vi "FRCts20_WebMethods_Division_DELETE.vi"(7 "httpRequestID":u32, 10 "division":string, 11 "competition":string) -> ()   [LabVIEW 2014, in "FRCts20_WebMethods.lvlib"]
doc: "<B>DELETE</B> the specified <B>division</B> resource\n\nhttp://<server address>:<port>/FRCts/competition/<B>competition</B>/division/<B>division</B>\n\n{requires authentication}"
uses:
  FRCts20_WebMethods.lvlib
  <vilib>/wsapi/NI_WebServices.lvlib
  Backend/source/VI Source/FRCts20_Backend_API/FRCts20_Backend_API_SW.ctl
  Backend/source/VI Source/FRCts20_Backend_API/FRCts20_Backend_API.lvlib
  Backend/source/VI Source/FRCts20_Backend_API/FRCts20_Backend_API_Status.ctl
  Backend/source/VI Source/FRCts20_Backend_API/FRCts20_Backend_API_Division.ctl
  Backend/source/VI Source/FRCts20_Backend_API/FRCts20_Backend_API_Command_Division.ctl
  Backend/source/VI Source/FRCts20_Backend_API/FRCts20_Backend_API_Application.vi
panel:
  in  "query":string
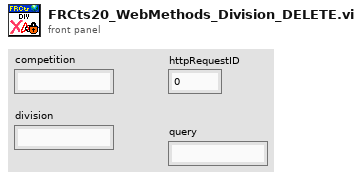
[diagram p1: front panel]
types:
  T1 = typedef "FRCts20_Backend_API.lvlib/FRCts20_Backend_API_Command_Division.ctl" = string
  T2 = typedef "FRCts20_Backend_API.lvlib/FRCts20_Backend_API_Division.ctl" = cluster{"Location":string, "Team":u32[], "APIReturn":string, "RootCmd":enum16{"Issues", "Software", "All"}, "SWType":T3, "Status":T4, "Competition":string}
  T3 = typedef "FRCts20_Backend_API.lvlib/FRCts20_Backend_API_SW.ctl" = string
  T4 = typedef "FRCts20_Backend_API.lvlib/FRCts20_Backend_API_Status.ctl" = enum16{"Open", "In Work", "Closed"}
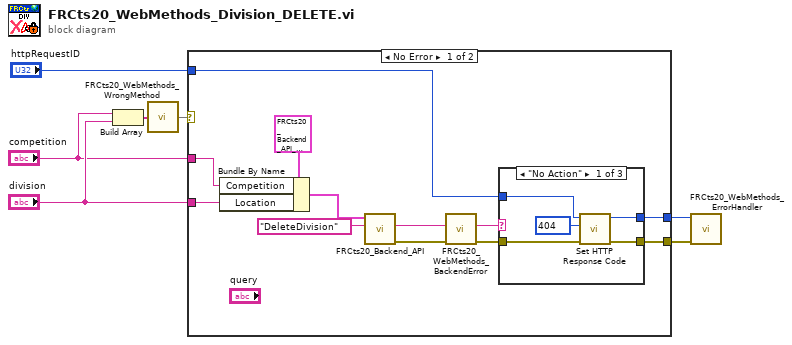
[diagram p0: block diagram]
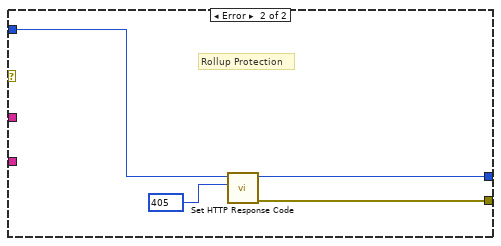
[diagram p4: hidden frame]
diagram:
  n1 = Build Array("competition", "division") -> (w6:string[])
  n2 = call "FRCts20_WebMethods_WrongMethod.vi"(4:w6) -> (1:w7)  [unwired: 3 in, 1 out]
  n3 = case shown="No Error" w7 {
    tunnel: "httpRequestID" -> [w9 w32]
    tunnel: [w8 w30] -> w3
    tunnel: [w10 w29] -> w4
    tunnel: "division" -> [w18 _]
    tunnel: "competition" -> [w17 _]
    frame No Error {
      n4 = Bundle By Name(cluster=T2 {"Location"="", "Team"=[], "APIReturn"="", "RootCmd"=enum."Issues", "SWType"="", "Status"=enum."Open", "Competition"=""} ("Division"), "Competition"=w17, "Location"=w18) -> (w16:T2)
      n5 = call-poly "FRCts20_Backend_API.vi"("Command"=T1 "DeleteDivision", 11:w16) -> ("error out"=w14:errorcluster, "Status"=w13:string)  [unwired: 7 in, 1 out]
      n6 = call "FRCts20_WebMethods_BackendError.vi"("error in (no error)"=w14, "Status"=w13) -> ("error out"=w11:errorcluster, "Status out"=w12:string)  [unwired: 8 in]
      n7 = case shown="\"No Action\"" w12 {
        tunnel: w11 -> [w21 w26 w28]
        tunnel: [w24 w26 w28] -> w10
        tunnel: w9 -> [w22 w25 w27]
        tunnel: [w23 w25 w27] -> w8
        frame "No Action" {
          w20 = 404 items=["100"=100, "101"=101, "200"=200, "201"=201, "202"=202, "203"=203, "204"=204, "205"=205, "206"=206, "300"=300, "301"=301, "302"=302, "303"=303, "304"=304, "305"=305, "306"=306, "307"=307, "400"=400, "401"=401, "402"=402, "403"=403, "404"=404, "405"=405, "406"=406, "407"=407, "408"=408, "409"=409, "410"=410, "411"=411, "412"=412, "413"=413, "414"=414, "415"=415, "416"=416, "417"=417, "500"=500, "501"=501, "502"=502, "503"=503, "504"=504, "505"=505] ("response code (200)")
          n8 = call <vilib>:"Set HTTP Response Code.vi"("error in (no error)"=w21, "response code (200)"=w20, "httpRequestID"=w22) -> ("error out"=w24:errorcluster, "httpRequestID out"=w23:u32)  [unwired: 7 in]
        }
        frame "Backend Error", Default {
        }
        frame "Success" {
        }
      }
    }
    frame Error {
      w31 = 405 items=["100"=100, "101"=101, "200"=200, "201"=201, "202"=202, "203"=203, "204"=204, "205"=205, "206"=206, "300"=300, "301"=301, "302"=302, "303"=303, "304"=304, "305"=305, "306"=306, "307"=307, "400"=400, "401"=401, "402"=402, "403"=403, "404"=404, "405"=405, "406"=406, "407"=407, "408"=408, "409"=409, "410"=410, "411"=411, "412"=412, "413"=413, "414"=414, "415"=415, "416"=416, "417"=417, "500"=500, "501"=501, "502"=502, "503"=503, "504"=504, "505"=505] ("response code (200)")
      # "Rollup Protection"
      n9 = call <vilib>:"Set HTTP Response Code.vi"("response code (200)"=w31, "httpRequestID"=w32) -> ("error out"=w29:errorcluster, "httpRequestID out"=w30:u32)  [unwired: 8 in]
    }
  }
  n10 = call "FRCts20_WebMethods_ErrorHandler.vi"("error in"=w4, "httpRequestID"=w3) -> ()  [unwired: 9 in, 1 out]
